vi "emi_Close all Loops.vi"(7 "Close Loops(T)":bool=TRUE, 11 "error in (no error)":errorcluster) -> (15 "error out":errorcluster)   [LabVIEW 2011]
doc: "Sends teh signal to close all loops. The closing is polled by each loop, so may take some time. Performs regardless of error in."
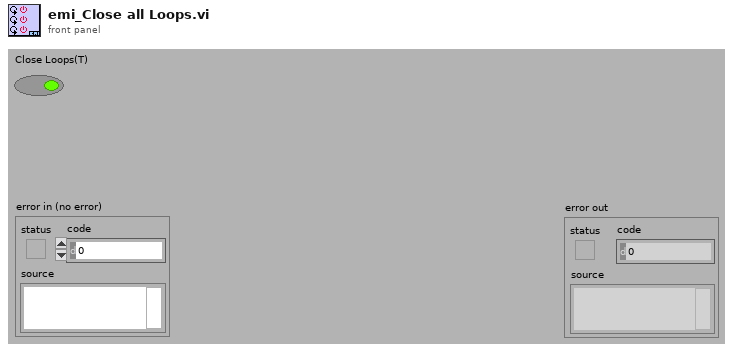
[diagram p1: front panel]
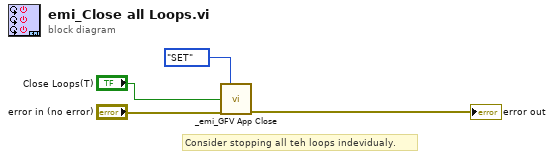
[diagram p0: block diagram]
diagram:
  # "Consider stopping all teh loops indevidualy."
  n1 = call "_emi_GFV App Close.vi"("Action(GET)"=enum16{"GET", "SET"}."SET", "App Close in"="Close Loops(T)", "error in (no error)"="error in (no error)") -> ("error out"=→"error out":errorcluster)  [unwired: 11 in, 1 out]
